vi "PreChecks.vi"(8 "type":T1(ring), 9 "Y":dbl, 11 "X":dbl) -> (1 "message":string, 3 "Error":bool)   [LabVIEW 2014]
uses:
  <userlib>/Nanonis Prog Interface V5/Scan/Piezos/Piezo Calibration Range Get.vi
  <userlib>/Nanonis Prog Interface V5/Nanonis Prog Interface.lvlib
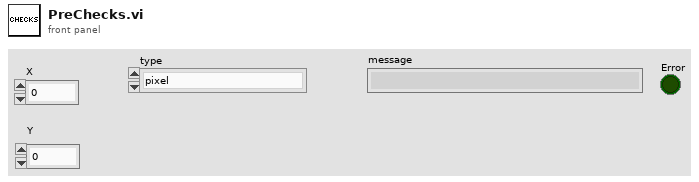
[diagram p1: front panel]
types:
  T1 = enum16{"pixel", "position", "size", "dip", "bias", "timing"}
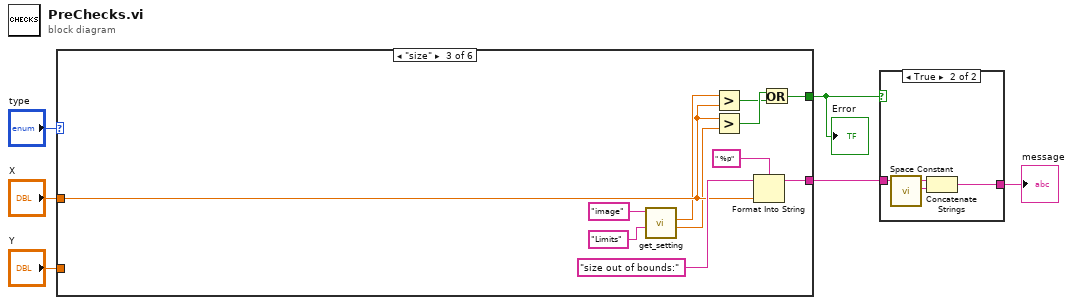
[diagram p0: block diagram]
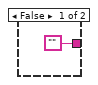
[diagram p2: hidden frame]
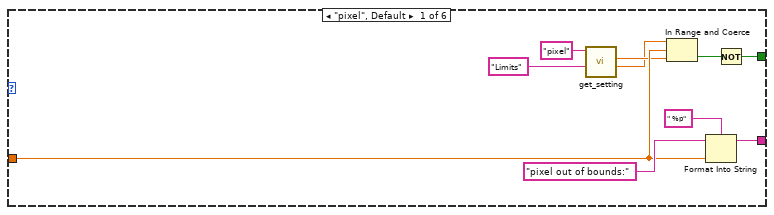
[diagram p3: hidden frame]
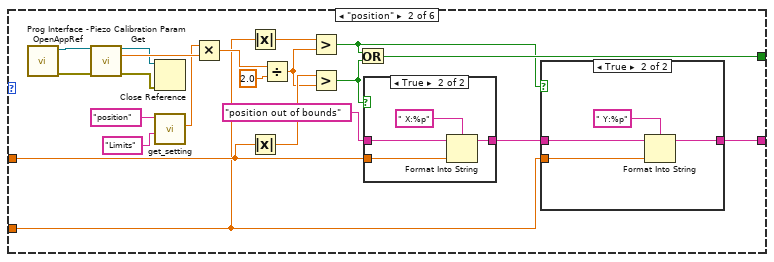
[diagram p4: hidden frame]
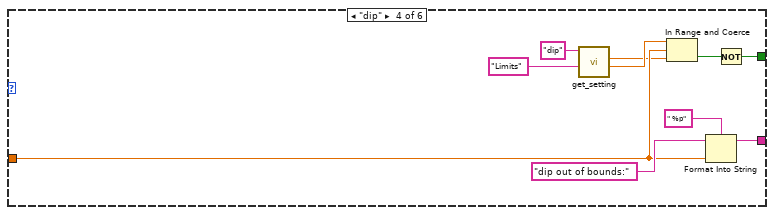
[diagram p7: hidden frame]
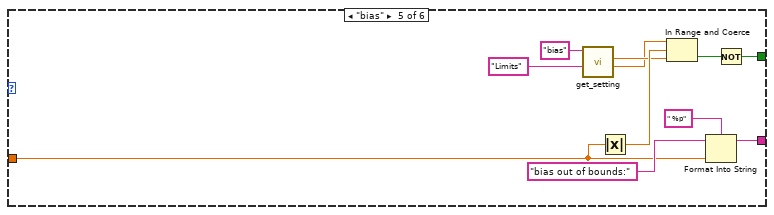
[diagram p8: hidden frame]
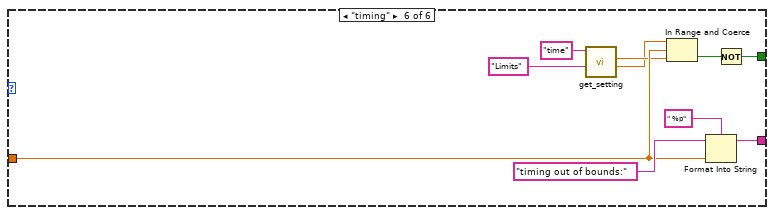
[diagram p9: hidden frame]
diagram:
  n1 = case shown="\"size\"" "type" {
    tunnel: "X" -> [w11 w26 w53 w63 w74 w84]
    tunnel: "Y" -> [_ w25 _ _ _ _]
    tunnel: [w15 w32 w56 w65 w78 w85] -> w3
    tunnel: [w12 w24 w52 w64 w75 w87] -> w2
    frame "pixel", Default {
      n2 = call "get_setting.vi"("section"="Limits", "key"="pixel") -> ("output 2"=w7:dbl, "output 1"=w8:dbl)  [unwired: 5 in, 3 out]
      n3 = In Range and Coerce(upper limit=w7, x=w11, lower limit=w8) -> (In Range?=w16:bool)  [unwired: 1 out]
      n4 = Format Into String(format string=" %p", initial string="pixel out of bounds:" ("message"), w11) -> (resulting string=w12:string)  [unwired: 1 in, 1 out]
      n5 = Not(x=w16) -> (.not. x?=w15:bool)
    }
    frame "position" {
      n6 = call <userlib>:"Prog Interface - OpenAppRef.vi"() -> ("Error out"=w20:errorcluster, "Application reference"=w21:refnum<vi>)  [unwired: 6 in]
      n7 = call-poly <userlib>:"Piezo Calibration Param Get.vi"("Application ref in"=w21, "error in (no error)"=w20) -> ("Application ref out"=w23:refnum<vi>, "Range X (m)"=w31:sgl, "error out"=w22:errorcluster)  [unwired: 9 in, 2 out]
      n8 = Close Reference(reference=w23, error in (no error)=w22) -> ()  [unwired: 1 out]
      n9 = call "get_setting.vi"("section"="Limits", "key"="position") -> ("output 1"=w17:dbl)  [unwired: 5 in, 4 out]
      n10 = Multiply(x=w17, y=w31) -> (x*y=w37:dbl)
      n11 = Absolute Value(x=w25) -> (abs(x)=w35:dbl)
      n12 = Absolute Value(x=w26) -> (abs(x)=w34:dbl)
      n13 = Divide(x=w37, y=2.0) -> (x/y=w33:dbl)
      n14 = Greater?(x=w35, y=w33) -> (0:w27:bool)
      n15 = Greater?(x=w34, y=w33) -> (0:w28:bool)
      n16 = Or(x=w27, y=w28) -> (x .or. y?=w32:bool)
      n17 = case shown="True" w28 {
        tunnel: "position out of bounds" ("message") -> [w43 w46]
        tunnel: [w43 w45] -> w29
        tunnel: w26 -> [_ w44]
        frame False {
        }
        frame True {
          n18 = Format Into String(format string=" X:%p", initial string=w46, w44) -> (resulting string=w45:string)  [unwired: 1 in, 1 out]
        }
      }
      n19 = case shown="True" w27 {
        tunnel: w29 -> [w38 w42]
        tunnel: w25 -> [_ w40]
        tunnel: [w38 w39] -> w24
        frame False {
        }
        frame True {
          n20 = Format Into String(format string=" Y:%p", initial string=w42, w40) -> (resulting string=w39:string)  [unwired: 1 in, 1 out]
        }
      }
    }
    frame "size" {
      n21 = call "get_setting.vi"("section"="Limits", "key"="image") -> ("output 2"=w48:dbl, "output 1"=w49:dbl)  [unwired: 5 in, 3 out]
      n22 = Greater?(x=w49, y=w53) -> (0:w57:bool)
      n23 = Greater?(x=w53, y=w48) -> (0:w58:bool)
      n24 = Format Into String(format string=" %p", initial string="size out of bounds:" ("message"), w53) -> (resulting string=w52:string)  [unwired: 1 in, 1 out]
      n25 = Or(x=w58, y=w57) -> (x .or. y?=w56:bool)
    }
    frame "dip" {
      n26 = call "get_setting.vi"("section"="Limits", "key"="dip") -> ("output 2"=w60:dbl, "output 1"=w59:dbl)  [unwired: 5 in, 3 out]
      n27 = In Range and Coerce(upper limit=w60, x=w63, lower limit=w59) -> (In Range?=w66:bool)  [unwired: 1 out]
      n28 = Format Into String(format string=" %p", initial string="dip out of bounds:" ("message"), w63) -> (resulting string=w64:string)  [unwired: 1 in, 1 out]
      n29 = Not(x=w66) -> (.not. x?=w65:bool)
    }
    frame "bias" {
      n30 = call "get_setting.vi"("section"="Limits", "key"="bias") -> ("output 2"=w69:dbl, "output 1"=w70:dbl)  [unwired: 5 in, 3 out]
      n31 = Absolute Value(x=w74) -> (abs(x)=w73:dbl)
      n32 = In Range and Coerce(upper limit=w69, x=w73, lower limit=w70) -> (In Range?=w79:bool)  [unwired: 1 out]
      n33 = Format Into String(format string=" %p", initial string="bias out of bounds:" ("message"), w74) -> (resulting string=w75:string)  [unwired: 1 in, 1 out]
      n34 = Not(x=w79) -> (.not. x?=w78:bool)
    }
    frame "timing" {
      n35 = call "get_setting.vi"("section"="Limits", "key"="time") -> ("output 2"=w80:dbl, "output 1"=w81:dbl)  [unwired: 5 in, 3 out]
      n36 = In Range and Coerce(upper limit=w80, x=w84, lower limit=w81) -> (In Range?=w86:bool)  [unwired: 1 out]
      n37 = Format Into String(format string=" %p", initial string="timing out of bounds:" ("message"), w84) -> (resulting string=w87:string)  [unwired: 1 in, 1 out]
      n38 = Not(x=w86) -> (.not. x?=w85:bool)
    }
  }
  "Error" <- w3
  n39 = case shown="True" w3 {
    tunnel: ["" w92] -> w1
    tunnel: w2 -> [_ w93]
    frame False {
    }
    frame True {
      n40 = call <vilib>:"Space Constant.vi"() -> ("String"=w91:string)
      n41 = Concatenate Strings(w93, w91) -> (w92:string)
    }
  }
  "message" <- w1
